vi "Ch1-32_Save_file_header.vi"(0 "File name":string="Name", 1 "Save":bool) -> (2 "Output Path":path)   [LabVIEW 2018]
uses:
  <vilib>/Utility/file.llb/Write To Spreadsheet File (string).vi
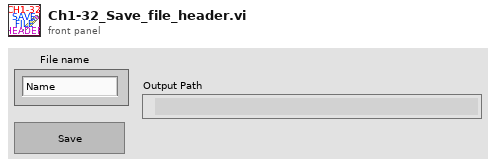
[diagram p1: front panel]
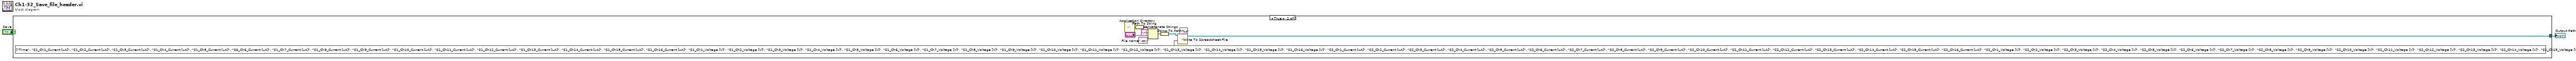
[diagram p0: block diagram]
diagram:
  n1 = case shown="True" "Save" {
    tunnel: [_ w3] -> w1
    frame False {
    }
    frame True {
      n2 = call <vilib>:"Application Directory.vi"() -> ("Application Directory"=w8:path)
      n3 = Path To String(path=w8) -> (string=w7:string)
      n4 = Concatenate Strings(w7, "/" ("string"), "File name", ".csv" ("string")) -> (w12:string)
      n5 = String To Path(string=w12) -> (path=w4:path)
      n6 = call-poly <vilib>:"Write To Spreadsheet File.vi"("format (%s)"="%s", "1D data"=string[] ["Time", "S1_Ch1_Current [uA]", "S1_Ch2_Current [uA]", "S1_Ch3_Current [uA]", "S1_Ch4_Current [uA]", "S1_Ch5_Current [uA]", "S6_Ch6_Current [uA]", "S1_Ch7_Current [uA]", "S1_Ch8_Current [uA]", "S1_Ch9_Current [uA]", "S1_Ch10_Current [uA]", "S1_Ch11_Current [uA]", "S1_Ch12_Current [uA]", "S1_Ch13_Current [uA]", "S1_Ch14_Current [uA]", "S1_Ch15_Current [uA]", "S1_Ch16_Current [uA]", "S1_Ch1_Voltage [V]", "S1_Ch2_Voltage [V]", "S1_Ch3_Voltage [V]", "S1_Ch4_Voltage [V]", "S1_Ch5_Voltage [V]", "S1_Ch6_Voltage [V]", "S1_Ch7_Voltage [V]", "S1_Ch8_Voltage [V]", "S1_Ch9_Voltage [V]", "S1_Ch10_Voltage [V]", "S1_Ch11_Voltage [V]", "S1_Ch12_Voltage [V]", "S1_Ch13_Voltage [V]", "S1_Ch14_Voltage [V]", "S1_Ch15_Voltage [V]", "S1_Ch16_Voltage [V]", "S2_Ch1_Current [uA]", "S2_Ch2_Current [uA]", "S2_Ch3_Current [uA]", "S2_Ch4_Current [uA]", "S2_Ch5_Current [uA]", "S2_Ch6_Current [uA]", "S2_Ch7_Current [uA]", "S2_Ch8_Current [uA]", "S2_Ch9_Current [uA]", "S2_Ch10_Current [uA]", "S2_Ch11_Current [uA]", "S2_Ch12_Current [uA]", "S2_Ch13_Current [uA]", "S2_Ch14_Current [uA]", "S2_Ch15_Current [uA]", "S2_Ch16_Current [uA]", "S2_Ch1_Voltage [V]", "S2_Ch2_Voltage [V]", "S2_Ch3_Voltage [V]", "S2_Ch4_Voltage [V]", "S2_Ch5_Voltage [V]", "S2_Ch6_Voltage [V]", "S2_Ch7_Voltage [V]", "S2_Ch8_Voltage [V]", "S2_Ch9_Voltage [V]", "S2_Ch10_Voltage [V]", "S2_Ch11_Voltage [V]", "S2_Ch12_Voltage [V]", "S2_Ch13_Voltage [V]", "S2_Ch14_Voltage [V]", "S2_Ch15_Voltage [V]", "S2_Ch16_Voltage [V]"], "file path (dialog if empty)"=w4) -> ("new file path (Not A Path if cancelled)"=w3:path)  [unwired: 5 in]
    }
  }
  "Output Path" <- w1
